vi "set_speed_params.vi"(6 "pixel-dwell time":dbl[unit]=-1.0, 7 "speed param":T1, 8 "error in (no error)":errorcluster, 9 "line-scan time":dbl[unit]=-1.0, 10 "frame rate":dbl[unit]=-1.0, 11 "TrajectoryDL090201FrameScan in":refnum<class "TrajectoryDL090201FrameScan.lvclass">) -> (0 "error out":errorcluster, 3 "TrajectoryDL090201FrameScan out":refnum<class "TrajectoryDL090201FrameScan.lvclass">)   [LabVIEW 2010, in "TrajectoryDL090201FrameScan.lvclass"]
uses:
  TrajectoryDL090201FrameScan.lvclass
  speed_param_enum.ctl
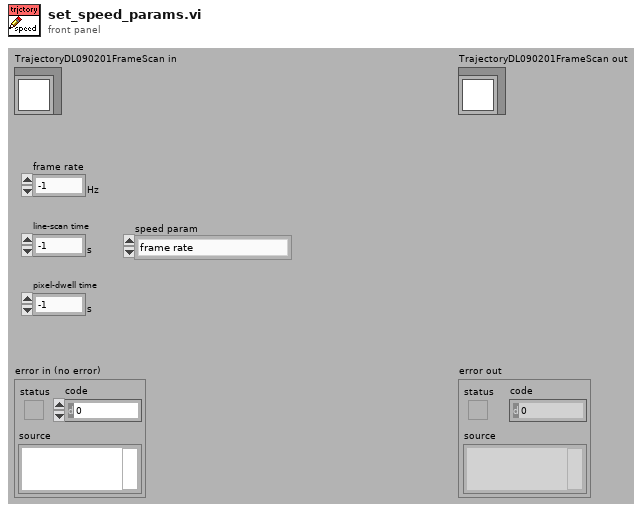
[diagram p1: front panel]
types:
  T1 = typedef "TrajectoryDL090201FrameScan.lvclass/speed_param_enum.ctl" = enum16{"frame rate", "line-scan time", "pixel-dwell time"}
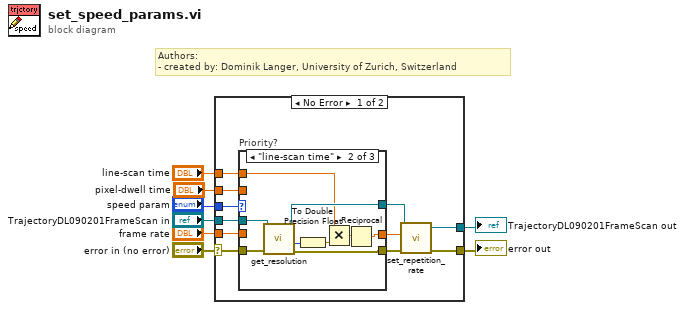
[diagram p0: block diagram]
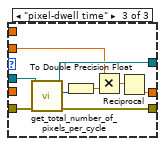
[diagram p3: hidden frame]
diagram:
  # "Authors: \n- created by: Dominik Langer, University of Zurich, Switzerland"
  n1 = case shown="No Error" "error in (no error)" {
    selector: "error in (no error)" -> [w17 w42]
    tunnel: [w19 w42] -> w7
    tunnel: [w13 w41] -> w5
    tunnel: "TrajectoryDL090201FrameScan in" -> [w10 w41]
    tunnel: "speed param" -> [w18 _]
    tunnel: "pixel-dwell time" -> [w11 _]
    tunnel: "line-scan time" -> [w12 _]
    tunnel: "frame rate" -> [w16 _]
    frame No Error {
      n2 = case "Priority?" shown="\"line-scan time\"" w18 {
        tunnel: w17 -> [w22 w31 w40]
        tunnel: w16 -> [w21 _ _]
        tunnel: [w22 w28 w37] -> w15
        tunnel: [w21 w23 w32] -> w14
        tunnel: w12 -> [_ w26 _]
        tunnel: w11 -> [_ _ w34]
        tunnel: w10 -> [w20 w30 w39]
        tunnel: [w20 w27 w38] -> w9
        frame "frame rate", Default {
        }
        frame "line-scan time" {
          n3 = call-dynamic "get_resolution.vi"("error in (no error)"=w31, "TrajectoryDL090201FrameScan in"=w30) -> ("error out"=w28:errorcluster, "y"=w29:i32, "TrajectoryDL090201FrameScan out"=w27:refnum<class "TrajectoryDL090201FrameScan.lvclass">)  [unwired: 6 in, 1 out]
          n4 = To Double Precision Float(number=w29) -> (double precision float=w25:dbl)
          n5 = Multiply(x=w26, y=w25) -> (x*y=w24:dbl[unit])
          n6 = Reciprocal(x=w24) -> (1/x=w23:dbl[unit])
        }
        frame "pixel-dwell time" {
          n7 = call-dynamic "get_total_number_of_pixels_per_cycle.vi"("error in (no error)"=w40, "TrajectoryDL090201FrameScan in"=w39) -> ("error out"=w37:errorcluster, "total number of pixels per cycle"=w36:i32, "TrajectoryDL090201FrameScan out"=w38:refnum<class "TrajectoryDL090201FrameScan.lvclass">)  [unwired: 7 in]
          n8 = To Double Precision Float(number=w36) -> (double precision float=w35:dbl)
          n9 = Multiply(x=w34, y=w35) -> (x*y=w33:dbl[unit])
          n10 = Reciprocal(x=w33) -> (1/x=w32:dbl[unit])
        }
      }
      n11 = call-dynamic "set_repetition_rate.vi"("error in (no error)"=w15, "repetition rate"=w14, "GenericTrajectory in"=w9) -> ("error out"=w19:errorcluster, "GenericTrajectory out"=w13:refnum<class "TrajectoryDL090201FrameScan.lvclass">)  [unwired: 7 in]
    }
    frame Error {
    }
  }
  "error out" <- w7
  "TrajectoryDL090201FrameScan out" <- w5
